vi "Main.vi"   [LabVIEW 2011]
types:
  T1 = typedef "WPI_DriverStationRobotMode.ctl" = enum16{"Autonomous Disabled", "Autonomous Enabled", "Teleop Disabled", "Teleop Enabled", "Timeout", "Finish"}
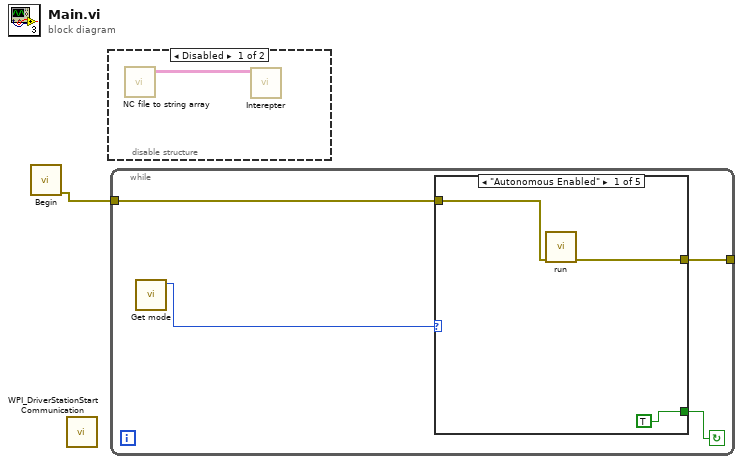
[diagram p0: block diagram]
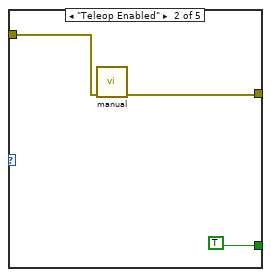
[diagram p2: hidden frame]
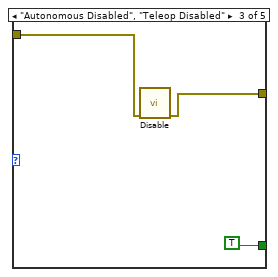
[diagram p3: hidden frame]
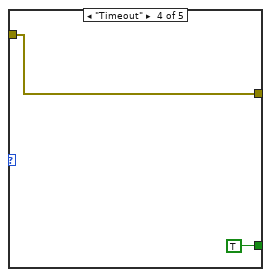
[diagram p4: hidden frame]
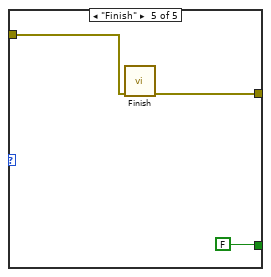
[diagram p5: hidden frame]
diagram:
  n1 = call "Begin.vi"() -> ("error out"=w1:errorcluster)  [unwired: 11 in]
  n2 = call <vilib>:"WPI_DriverStationStart Communication.vi"() -> ()  [unwired: 12 in]
  n3 = disable-structure shown="Disabled" {
    frame Disabled {
      n4 = call "NC file to string array.vi"() -> ("Code"=w2:string[][])  [unwired: 10 in, 1 out]
      n5 = call "Interepter.vi"("Array"=w2) -> ()  [unwired: 11 in]
    }
    frame Enabled {
    }
  }
  n6 = while {
    tunnel: w1 -> [w4]
    tunnel: [w3] -> _
    stop <- w5 continue-if-true
    n7 = call "Get mode.vi"() -> ("Robot Mode"=w6:T1)  [unwired: 11 in]
    n8 = case shown="\"Autonomous Enabled\"" w6 {
      tunnel: [TRUE TRUE TRUE TRUE FALSE] -> w5
      tunnel: w4 -> [w8 w11 w14 w16 w19]
      tunnel: [w7 w10 w13 w16 w18] -> w3
      frame "Autonomous Enabled" {
        n9 = call "run.vi"("error in (no error)"=w8) -> ("error out"=w7:errorcluster)  [unwired: 10 in]
      }
      frame "Teleop Enabled" {
        n10 = call "manual.vi"("error in (no error)"=w11) -> ("error out"=w10:errorcluster)  [unwired: 10 in]
      }
      frame "Autonomous Disabled", "Teleop Disabled" {
        n11 = call "Disable.vi"("error in (no error)"=w14) -> ("error out"=w13:errorcluster)  [unwired: 10 in]
      }
      frame "Timeout" {
      }
      frame "Finish" {
        n12 = call "Finish.vi"("error in (no error)"=w19) -> ("error out"=w18:errorcluster)  [unwired: 10 in]
      }
    }
  }
